vi "example.vi"() -> ()   [LabVIEW 2019]
panel:
  in  "List":i32[](array[numeric])=[0, 0, 0, 0, 0, 0, 0, 0, 0, 0]
  out "s? t:f":errorcluster
  in  "error in":errorcluster
  out "probability not equal to 1":bool
  in  "number of unique samples":i32
  out "samples":i32[](array[numeric])
  in  "probability":dbl[](array[numeric])
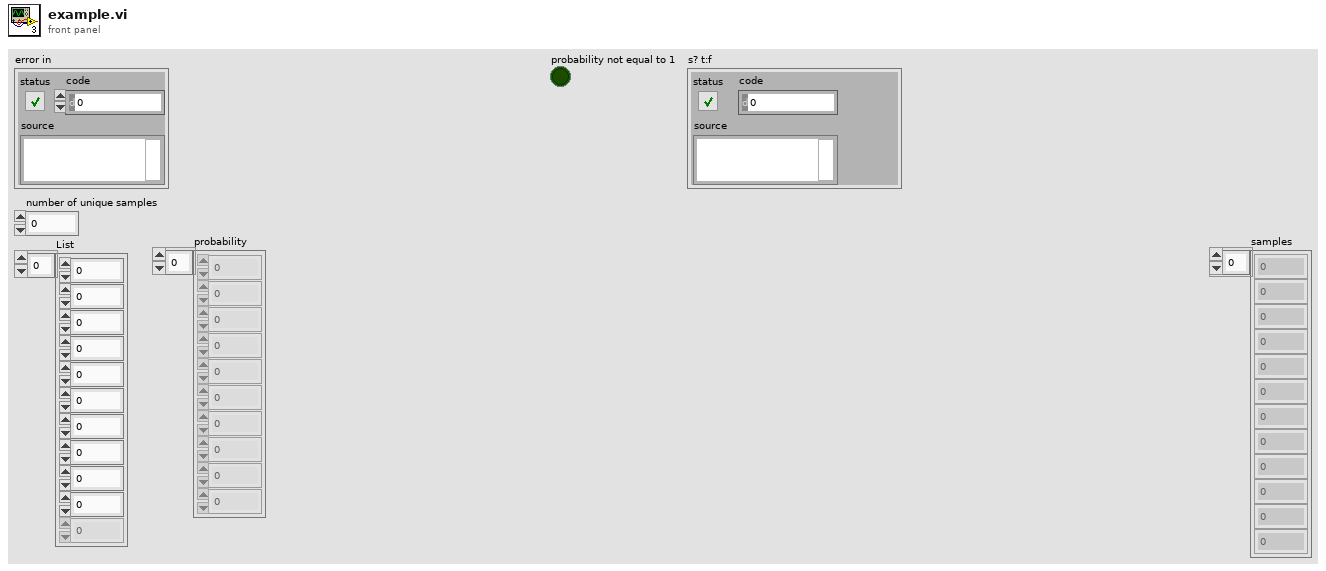
[diagram p1: front panel]
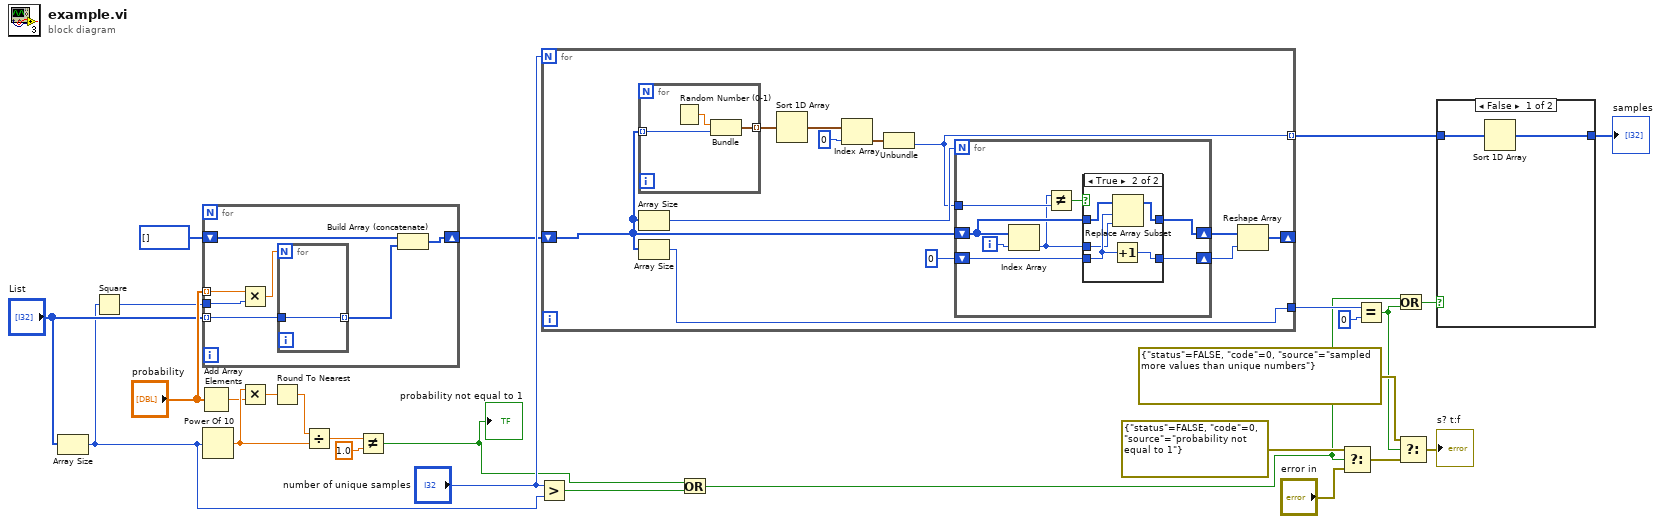
[diagram p0: block diagram]
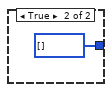
[diagram p2: hidden frame]
diagram:
  n1 = Array Size(array="List") -> (size(s)=w15:i32)
  n2 = Square(x=w15) -> (x^2=w20:i32)
  n3 = Add Array Elements(numeric array="probability") -> (sum=w21:dbl)
  n4 = for {
    tunnel: "probability" -> [w34] mode=indexing
    tunnel: "List" -> [w32] mode=indexing
    shift-right: [w30] -> w11
    shift-left: i32[] [] -> [w29]
    tunnel: w20 -> [w28]
    n5 = Multiply(x=w34, y=w28) -> (x*y=w33:dbl)
    n6 = for {
      N: w33 -> [_]
      tunnel: w32 -> [w35]
      tunnel: [w35] -> w31 mode=indexing
    }
    n7 = Build Array (concatenate)(w29, w31) -> (w30:i32[])
  }
  n8 = Power Of 10(x=w15) -> (10^x=w22:dbl)
  n9 = Multiply(x=w22, y=w21) -> (x*y=w24:dbl)
  n10 = Round To Nearest(number=w24) -> (nearest integer value=w23:dbl)
  n11 = Divide(x=w23, y=w22) -> (x/y=w19:dbl)
  n12 = Not Equal?(x=w19, y=1.0) -> (x != y?=w13:bool)
  "probability not equal to 1" <- w13
  n13 = Greater?(x="number of unique samples", y=w15) -> (0:w14:bool)
  n14 = for {
    N: "number of unique samples" -> [_]
    tunnel: [w39] -> w4 mode=indexing
    shift-right: [w38] -> _
    shift-left: w11 -> [w37]
    tunnel: [w36] -> w8
    n15 = for {
      tunnel: [w65] -> w47 mode=indexing
      tunnel: w37 -> [w63] mode=indexing
      n16 = Random Number (0-1)() -> (number: 0 to 1=w64:dbl)
      n17 = Bundle("number: 0 to 1"=w64, w63) -> (w65:cluster{"number: 0 to 1":dbl, i32})  [unwired: 1 out]
    }
    n18 = Array Size(array=w37) -> (size(s)=w43:i32)
    n19 = Array Size(array=w37) -> (size(s)=w36:i32)
    n20 = Sort 1D Array(array=w47) -> (sorted array=w46:cluster{"number: 0 to 1":dbl, i32}[])
    n21 = Index Array(array=w46, index=0) -> (element=w45:cluster{"number: 0 to 1":dbl, i32})
    n22 = Unbundle(w45) -> (w39:i32)  [unwired: 1 out]
    n23 = for {
      N: w43 -> [_]
      shift-right: [w55] -> w41
      shift-left: w37 -> [w53]
      shift-right: [w51] -> w40
      shift-left: 0 -> [w52]
      tunnel: w39 -> [w50]
      i -> [w54]
      n24 = Index Array(array=w53, index=w54) -> (element=w48:i32)
      n25 = Not Equal?(x=w48, y=w50) -> (x != y?=w49:bool)
      n26 = case shown="True" w49 {
        tunnel: w53 -> [w57 w62]
        tunnel: [w57 w61] -> w55
        tunnel: w52 -> [w56 w60]
        tunnel: [w56 w59] -> w51
        tunnel: w48 -> [_ w58]
        frame False {
        }
        frame True {
          n27 = Increment(x=w60) -> (x+1=w59:i32)
          n28 = Replace Array Subset(array=w62, new element=w58, index=w60) -> (w61:i32[])
        }
      }
    }
    n29 = Reshape Array(w41, w40) -> (w38:i32[])
  }
  n30 = Or(x=w13, y=w14) -> (x .or. y?=w3:bool)
  n31 = Select(t=errorcluster {"status"=FALSE, "code"=0, "source"="probability not equal to 1"} ("error constant"), s=w3, f="error in") -> (s? t:f=w6:errorcluster)
  n32 = Equal?(x=w8, y=0) -> (x = y?=w2:bool)
  n33 = Or(x=w3, y=w2) -> (x .or. y?=w1:bool)
  n34 = Select(t=errorcluster {"status"=FALSE, "code"=0, "source"="sampled more values than unique numbers"} ("error constant"), s=w2, f=w6) -> (s? t:f=→"s? t:f":errorcluster)
  n35 = case shown="False" w1 {
    tunnel: [w66 i32[] []] -> w5
    tunnel: w4 -> [w67 _]
    frame False {
      n36 = Sort 1D Array(array=w67) -> (sorted array=w66:i32[])
    }
    frame True {
    }
  }
  "samples" <- w5
